vi "Read_Joint_States_Notifier.vi"(4 "Side":T1=enum."right", 5 "error in":errorcluster, 8 "ignore previous (F)":bool) -> (0 "error out":errorcluster, 3 "Positions":dbl[](array[numeric]) format="%.3f")   [LabVIEW 2013]
uses:
  ROS/Code/SubVIs/BaxterSide.ctl
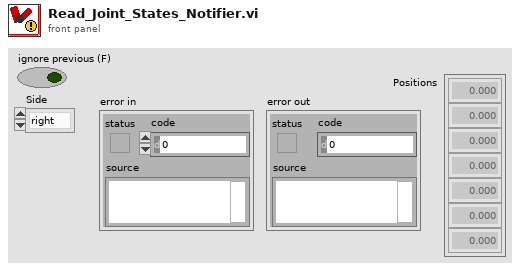
[diagram p1: front panel]
types:
  T1 = typedef "BaxterSide.ctl" = enum16{"left", "right"}
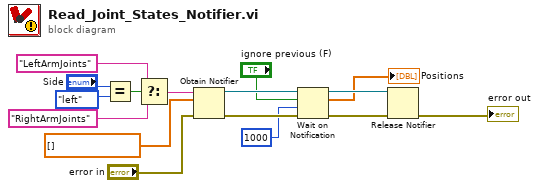
[diagram p0: block diagram]
diagram:
  n1 = Equal?(x="Side", y=BaxterSide."left" ("Side")) -> (x = y?=w5:bool)
  n2 = Select(t="LeftArmJoints", s=w5, f="RightArmJoints") -> (s? t:f=w16:string)
  n3 = Obtain Notifier(name (unnamed)=w16, notification data type=dbl[] [], error in (no error)="error in") -> (notifier out=w12:refnum<notifier>, error out=w7:errorcluster)  [unwired: 1 in, 1 out]
  n4 = Wait on Notification(notifier=w12, ignore previous (F)="ignore previous (F)", timeout in ms (-1)=1000, error in (no error)=w7) -> (notifier out=w10:refnum<notifier>, notification=→"Positions":dbl[], error out=w8:errorcluster)  [unwired: 1 out]
  n5 = Release Notifier(notifier=w10, error in (no error)=w8) -> (error out=→"error out":errorcluster)  [unwired: 1 in, 2 out]
